vi "Convert_String_Data_to_Int_totals.vi"(1 "Province Data Out":string[][](array[string])) -> (0 "Array":i32[](array[numeric]))   [LabVIEW 2015]
doc: "Converts the filtered 2D string array into a 1D integer array with the daily data."
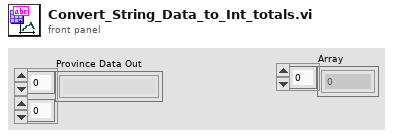
[diagram p1: front panel]
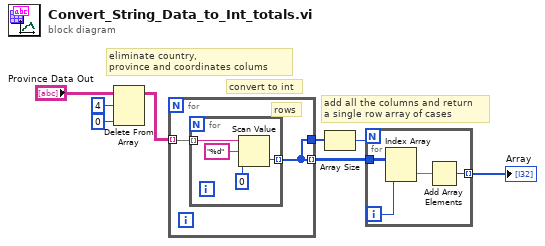
[diagram p0: block diagram]
diagram:
  # "add all the columns and return\na single row array of cases"
  # "convert to int"
  # "eliminate country,\nprovince and coordinates colums"
  n1 = Delete From Array(array="Province Data Out", length=4, index (col)=0 ("disabled index (col)")) -> (array with subset deleted=w4:string[][])  [unwired: 1 in, 1 out]
  n2 = for {
    tunnel: w4 -> [w10] mode=indexing
    tunnel: [w9] -> w5 mode=indexing
    tunnel: [w9] -> w6
    # "rows"
    n3 = for {
      tunnel: w10 -> [w14] mode=indexing
      tunnel: [w11] -> w9 mode=indexing
      n4 = Scan Value(string=w14, format string="%d", default (0 dbl)=0 ("disabled index (col)")) -> (value=w11:i32)  [unwired: 1 out]
    }
  }
  n5 = Array Size(array=w6) -> (size(s)=w7:i32)
  n6 = for {
    N: w7 -> [_]
    tunnel: w5 -> [w18]
    tunnel: [w15] -> w8 mode=indexing
    i -> [w17]
    n7 = Index Array(array=w18, index (col)=w17) -> (element=w16:i32[])  [unwired: 1 in]
    n8 = Add Array Elements(numeric array=w16) -> (sum=w15:i32)
  }
  "Array" <- w8
